vi "Load States.vi"(5 "Debug":T1, 6 "Constants":refnum<class "Sequence Constants.lvclass">, 7 "Seq Name":string, 8 "error in":refnum<class "MultiErrors.lvclass">, 10 "Config Element":refnum<class "Config Element.lvclass">) -> (0 "error out":refnum<class "MultiErrors.lvclass">, 2 "States":map{string, T2}(c390))   [LabVIEW 2023, in "VolatusSeqConfig.lvlib" / "Sequence Config.lvclass"]
uses:
  Sequence Config.lvclass
  lv-cdm/CDM-Config/Config Element/Config Element.lvclass
  State.ctl
  Step.ctl
  VolatusErrorUtilities/MultiErrors/MultiErrors.lvclass
  Sequence Constants/Sequence Constants.lvclass
  VolatusErrorUtilities/MultiErrors/MultiErrors.lvclass/MultiErrors.ctl
  Sequence Config.lvclass/Sequence Config.ctl
  Transition Config/Transition Config.lvclass
  Command Config/Command Config.lvclass
  VolatusSeqConfig.lvlib
  Debug Flags.ctl
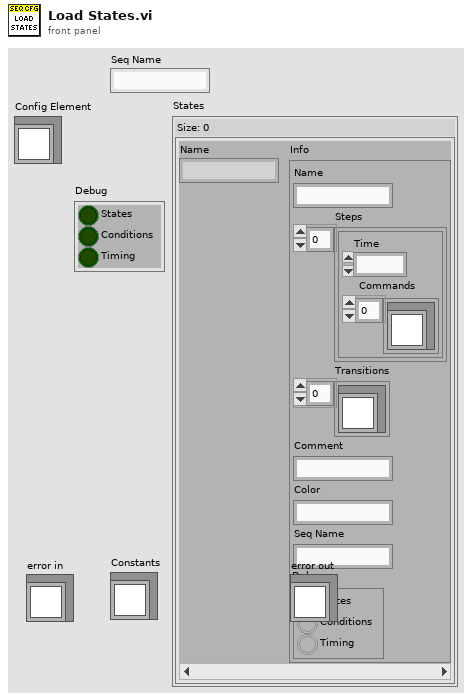
[diagram p1: front panel]
types:
  T1 = typedef "VolatusSeqConfig.lvlib/Debug Flags.ctl" = cluster{"States":bool, "Conditions":bool, "Timing":bool}
  T2 = typedef "VolatusSeqConfig.lvlib/State.ctl" = cluster{"Name":string, "Steps":T3[], "Transitions":refnum<class "Transition Config.lvclass">[], "Comment":string, "Color":string, "Seq Name":string, "Debug":T1}
  T3 = typedef "VolatusSeqConfig.lvlib/Step.ctl" = cluster{"Time":dbl, "Commands":refnum<class "Command Config.lvclass">[]}
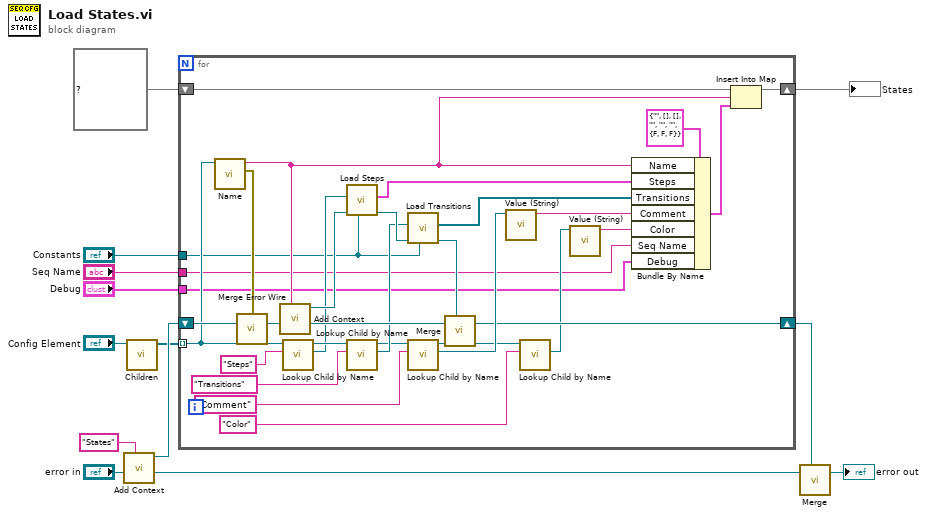
[diagram p0: block diagram]
diagram:
  n1 = call "Add Context.vi"("Context"="States", "MultiErrors in"="error in") -> ("Original Context"=w6:refnum<class "MultiErrors.lvclass">, "Added Context"=w13:refnum<class "MultiErrors.lvclass">)  [unwired: 8 in]
  n2 = call "Children.vi"("Config Element in"="Config Element") -> ("Elements"=w11:refnum<class "Config Element.lvclass">[])  [unwired: 9 in, 1 out]
  n3 = for {
    tunnel: w11 -> [w26] mode=indexing
    shift-right: [w31] -> w9
    shift-left: map{string, T2} {} ("States") -> [w33]
    shift-right: [w21] -> w4
    shift-left: w13 -> [w42]
    tunnel: "Constants" -> [w16]
    tunnel: "Seq Name" -> [w15]
    tunnel: "Debug" -> [w14]
    n4 = call "Name.vi"("Config Element in"=w26) -> ("error out"=w24:errorcluster, "Name"=w23:string)  [unwired: 9 in]
    n5 = call "Merge Error Wire.vi"("error in (no error)"=w24, "MultiErrors in"=w42) -> ("MultiErrors out"=w25:refnum<class "MultiErrors.lvclass">)  [unwired: 13 in]
    n6 = call "Add Context.vi"("Context"=w23, "MultiErrors in"=w25) -> ("Original Context"=w45:refnum<class "MultiErrors.lvclass">, "Added Context"=w44:refnum<class "MultiErrors.lvclass">)  [unwired: 8 in]
    n7 = call "Lookup Child by Name.vi"("Name"="Steps", "Config Element in"=w26) -> ("Child"=w38:refnum<class "Config Element.lvclass">, "Config Element out"=w40:refnum<class "Config Element.lvclass">)  [unwired: 6 in, 2 out]
    n8 = call "Load Steps.vi"("Constants"=w16, "error in"=w44, "Config Element"=w38) -> ("error out"=w43:refnum<class "MultiErrors.lvclass">, "Steps"=w36:T3[])  [unwired: 7 in]
    n9 = call "Lookup Child by Name.vi"("Name"="Transitions", "Config Element in"=w40) -> ("Child"=w35:refnum<class "Config Element.lvclass">, "Config Element out"=w30:refnum<class "Config Element.lvclass">)  [unwired: 6 in, 2 out]
    n10 = call "Load Transitions.vi"("Constants"=w16, "error in"=w43, "Config Element"=w35) -> ("error out"=w22:refnum<class "MultiErrors.lvclass">, "Transitions"=w34:refnum<class "Transition Config.lvclass">[])  [unwired: 7 in]
    n11 = call "Lookup Child by Name.vi"("Name"="Comment", "Config Element in"=w30) -> ("Child"=w28:refnum<class "Config Element.lvclass">, "Config Element out"=w20:refnum<class "Config Element.lvclass">)  [unwired: 6 in, 2 out]
    n12 = call "Merge.vi"("First Error In"=w45, "Second Error In"=w22) -> ("MultiErrors out"=w21:refnum<class "MultiErrors.lvclass">)  [unwired: 5 in]
    n13 = call "Value (String).vi"("Config Element in"=w28) -> ("String Value"=w27:string)  [unwired: 9 in, 1 out]
    n14 = call "Lookup Child by Name.vi"("Name"="Color", "Config Element in"=w20) -> ("Child"=w17:refnum<class "Config Element.lvclass">)  [unwired: 6 in, 3 out]
    n15 = call "Value (String).vi"("Config Element in"=w17) -> ("String Value"=w18:string)  [unwired: 9 in, 1 out]
    n16 = Bundle By Name(cluster=T2 {"Name"="", "Steps"=[], "Transitions"=[], "Comment"="", "Color"="", "Seq Name"="", "Debug"={"States"=FALSE, "Conditions"=FALSE, "Timing"=FALSE}} ("State"), "Name"=w23, "Steps"=w36, "Transitions"=w34, "Comment"=w27, "Color"=w18, "Seq Name"=w15, "Debug"=w14) -> (w32:T2)
    n17 = Insert Into Map(map in=w33, key=w23, value=w32) -> (map out=w31:map{string, T2})  [unwired: 2 out]
  }
  "States" <- w9
  n18 = call "Merge.vi"("First Error In"=w6, "Second Error In"=w4) -> ("MultiErrors out"=→"error out":refnum<class "MultiErrors.lvclass">)  [unwired: 5 in]
